vi "IMAGENES_100X100.vi"() -> ()   [LabVIEW 2016]
panel:
  out "IMAGEN_ORIGINAL":picture
  in  "path to JPEG file":path
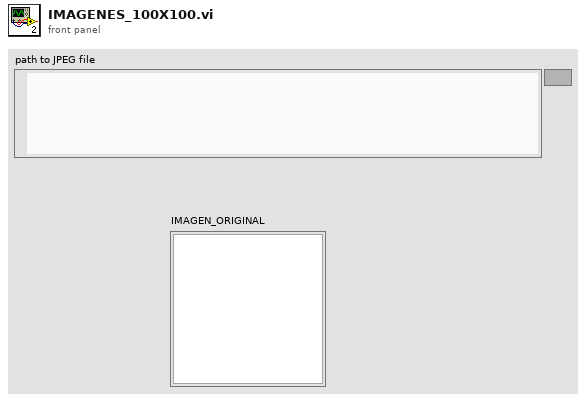
[diagram p1: front panel]
types:
  T1 = typedef "imagedata.ctl" = cluster{"image type":i32, "image depth":i32, "image":u8[], "mask":u8[], "colors":u32[], "Rectangle":cluster{"left":i16, "top":i16, "right":i16, "bottom":i16}}
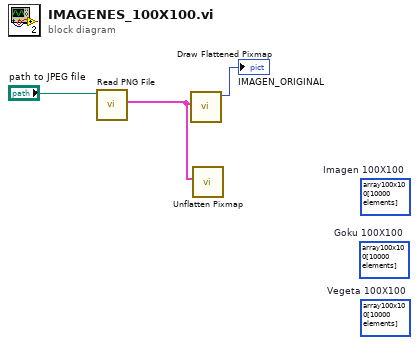
[diagram p0: block diagram]
diagram:
  (unwired) u32[][] array100x100[10000 elements]  # Vegeta 100X100
  (unwired) u32[][] array100x100[10000 elements]  # Goku 100X100
  (unwired) u32[][] array100x100[10000 elements]  # Imagen 100X100
  n1 = call <vilib>:"Read PNG File.vi"("path to PNG file"="path to JPEG file") -> ("image data"=w1:T1)  [unwired: 8 in, 2 out]
  n2 = call <vilib>:"Draw Flattened Pixmap.vi"("image data"=w1) -> ("new picture"=→"IMAGEN_ORIGINAL":picture)  [unwired: 8 in]
  n3 = call <vilib>:"Unflatten Pixmap.vi"("image data"=w1) -> ()  [unwired: 4 in, 7 out]
